vi "aal_Complex Modulator.vi"   [LabVIEW 2010, in "NI_AALPro.lvlib"]
uses:
  NI_AALPro.lvlib
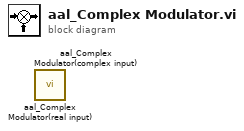
[diagram p0: block diagram]
diagram:
  n1 = call "aal_Complex Modulator(real input).vi"() -> ()  [unwired: 4 in, 1 out]
  n2 = call "aal_Complex Modulator(complex input).vi"() -> ()  [unwired: 4 in, 1 out]
